vi "niRFUtil WFM Detect Multiple Bursts (real wfm).vi"(0 "Waveform In (Ohm Voltage)":T2 {"y" min=0 max=127 format="%.2f"; "dx" format="%^.2e"; "x0" format="%^.2e"}, 5 "Burst Detection Settings":T1={"Mode"=enum."Sliding Window", "Sliding Window Settings"={"Chunks"=500, "Threshold (dB)"=12.0}, "Threshold Settings"={"Threshold Level (dB)"=-50.0, "Minimum Quiet Time (s)"=0.0001, "Threshold Type"=enum."Absolute"}} {"Threshold Settings"."Minimum Quiet Time (s)" format="%.3p"; "Threshold Settings"."Threshold Level (dB)" format="%.3g"; "Sliding Window Settings"."Threshold (dB)" format="%.3g"}) -> (4 "Number of Bursts Detected":i32, 6 "Burst Positions":cluster{"Start (s)":dbl, "Duration (s)":dbl}[](array[cluster]) {"Start (s)" format="%^.3e"; "Duration (s)" format="%^.3e"})   [LabVIEW 2015, in "niRFUtil.lvlib"]
uses:
  niRFUtil.lvlib
  Includes/niRFUtil INC Real Waveform.ctl
  Includes/niRFUtil INC Real Array.ctl
  Includes/niRFUtil INC Edge Detection Settings.ctl
  Includes/niRFUtil INC Edge Type.ctl
  niRFUtil WFM Detect Edge (complex wfm).vi
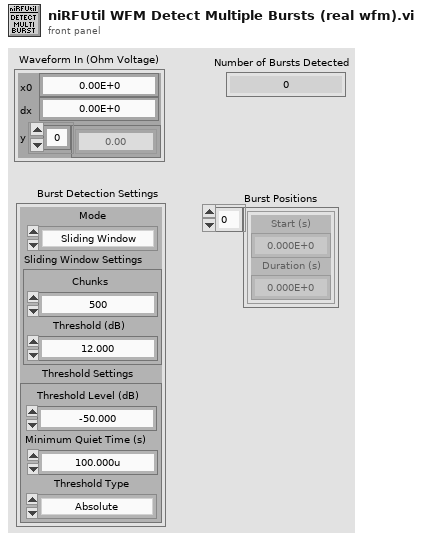
[diagram p1: front panel]
types:
  T1 = typedef "niRFUtil.lvlib/niRFUtil INC Edge Detection Settings.ctl" = cluster{"Mode":enum16{"Sliding Window", "Threshold"}, "Sliding Window Settings":cluster{"Chunks":i32, "Threshold (dB)":dbl}, "Threshold Settings":cluster{"Threshold Level (dB)":dbl, "Minimum Quiet Time (s)":dbl, "Threshold Type":enum16{"Relative", "Absolute"}}}
  T2 = typedef "niRFUtil.lvlib/niRFUtil INC Real Waveform.ctl" = cluster{"x0":dbl, "dx":dbl, "y":T3}
  T3 = typedef "niRFUtil.lvlib/niRFUtil INC Real Array.ctl" = sgl[]
  T4 = typedef "niRFUtil.lvlib/niRFUtil INC Edge Type.ctl" = enum16{"Rising", "Falling"}
  T5 = typedef "niRFUtil.lvlib/niRFUtil INC Complex Waveform.ctl" = cluster{"x0":dbl, "dx":dbl, "y":T6}
  T6 = typedef "niRFUtil.lvlib/niRFUtil INC Complex Array.ctl" = csg[]
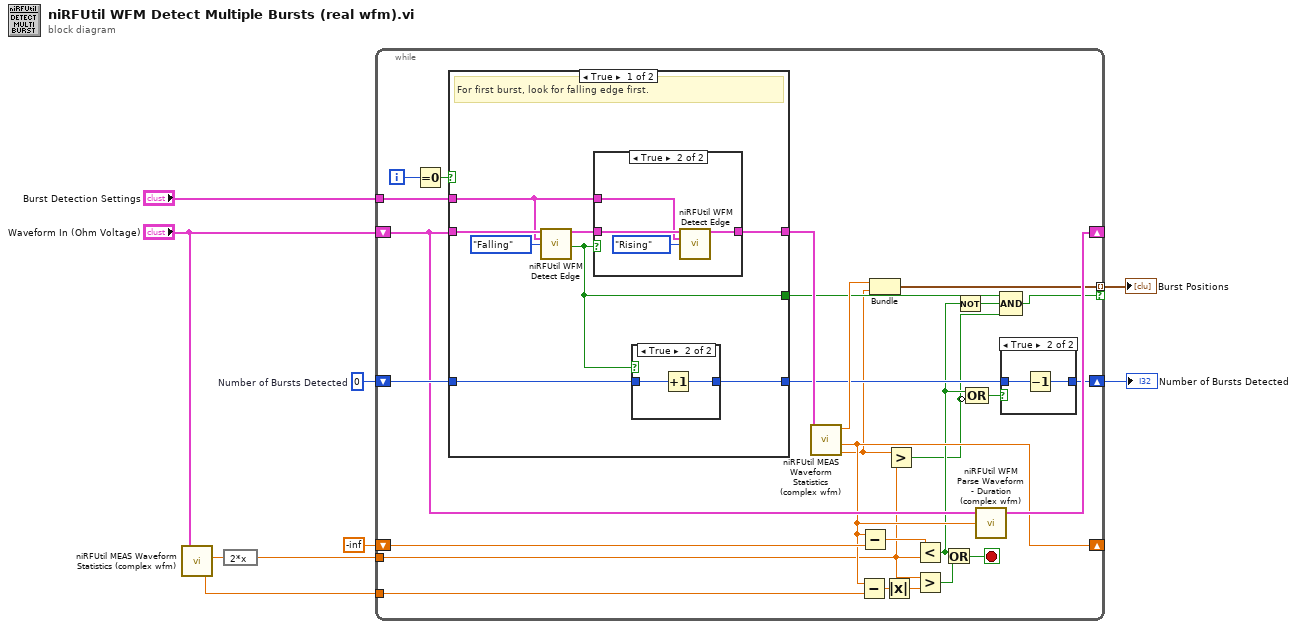
[diagram p0: block diagram]
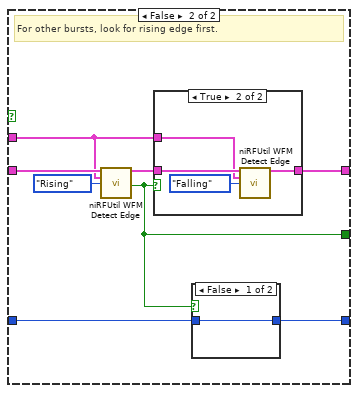
[diagram p5: hidden frame]
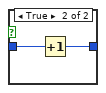
[diagram p6: hidden frame]
diagram:
  w9 = 0  # Number of Bursts Detected
  n1 = call "niRFUtil MEAS Waveform Statistics (complex wfm).vi"("Waveform In"="Waveform In (Ohm Voltage)") -> ("Interval"=w7:dbl, "End + Interval"=w5:dbl)  [unwired: 4 in, 2 out]
  n2 = expression code="2*x"(w7) -> (w6:dbl)
  n3 = while {
    shift-right: [w31] -> _
    shift-left: "Waveform In (Ohm Voltage)" -> [w33]
    shift-right: [w19] -> w4
    shift-left: w9 -> [w34]
    shift-right: [w22] -> _
    shift-left: -inf ("End") -> [w30]
    tunnel: w6 -> [w14]
    tunnel: w5 -> [w28]
    tunnel: [w21] -> w3 mode=indexing if=w16
    tunnel: "Burst Detection Settings" -> [w15]
    i -> [w36]
    stop <- w24 stop-if-true
    n4 = Equal To 0?(x=w36) -> (x = 0?=w35:bool)
    n5 = case shown="True" w35 {
      tunnel: w33 -> [w47 w63]
      tunnel: [w44 w60] -> w32
      tunnel: w34 -> [w43 w59]
      tunnel: [w42 w58] -> w20
      tunnel: [w41 w57] -> w17
      tunnel: w15 -> [w40 w56]
      frame True {
        # "For first burst, look for falling edge first."
        n6 = call-poly "niRFUtil WFM Detect Edge.vi"("Input Waveform"=w47, "Edge Detection Settings"=w40, "Edge Type"=niRFUtil_INC_Edge_Type."Falling") -> ("Output Waveform"=w45:T5, "Edge Detected?"=w41:bool)  [unwired: 9 in, 2 out]
        n7 = case shown="True" w41 {
          tunnel: w45 -> [w51 w55]
          tunnel: [w51 w53] -> w44
          tunnel: w40 -> [_ w52]
          frame False {
          }
          frame True {
            n8 = call-poly "niRFUtil WFM Detect Edge.vi"("Input Waveform"=w55, "Edge Detection Settings"=w52, "Edge Type"=niRFUtil_INC_Edge_Type."Rising") -> ("Output Waveform"=w53:T5)  [unwired: 9 in, 3 out]
          }
        }
        n9 = case shown="True" w41 {
          tunnel: w43 -> [w48 w50]
          tunnel: [w48 w49] -> w42
          frame False {
          }
          frame True {
            n10 = Increment(x=w50) -> (x+1=w49:i32)
          }
        }
      }
      frame False {
        # "For other bursts, look for rising edge first."
        n11 = call-poly "niRFUtil WFM Detect Edge.vi"("Input Waveform"=w63, "Edge Detection Settings"=w56, "Edge Type"=niRFUtil_INC_Edge_Type."Rising") -> ("Output Waveform"=w61:T5, "Edge Detected?"=w57:bool)  [unwired: 9 in, 2 out]
        n12 = case shown="True" w57 {
          tunnel: w61 -> [w67 w71]
          tunnel: [w67 w69] -> w60
          tunnel: w56 -> [_ w68]
          frame False {
          }
          frame True {
            n13 = call-poly "niRFUtil WFM Detect Edge.vi"("Input Waveform"=w71, "Edge Detection Settings"=w68, "Edge Type"=niRFUtil_INC_Edge_Type."Falling") -> ("Output Waveform"=w69:T5)  [unwired: 9 in, 3 out]
          }
        }
        n14 = case shown="False" w57 {
          tunnel: w59 -> [w64 w66]
          tunnel: [w64 w65] -> w58
          frame False {
          }
          frame True {
            n15 = Increment(x=w66) -> (x+1=w65:i32)
          }
        }
      }
    }
    n16 = call "niRFUtil MEAS Waveform Statistics (complex wfm).vi"("Waveform In"=w32) -> ("Start"=w23:dbl, "End + Interval"=w22:dbl, "Duration"=w10:dbl)  [unwired: 4 in, 1 out]
    n17 = Subtract(x=w22, y=w28) -> (x-y=w27:dbl)
    n18 = Subtract(x=w22, y=w30) -> (x-y=w29:dbl)
    n19 = Bundle("Start"=w23, "Duration"=w10) -> (w21:cluster{"Start":dbl, "Duration":dbl})  [unwired: 1 in]
    n20 = Absolute Value(x=w27) -> (abs(x)=w26:dbl)
    n21 = Greater?(x=w10, y=w14) -> (0:w11:bool)
    n22 = Less?(x=w29, y=w14) -> (x < y?=w13:bool)
    n23 = Greater?(x=w14, y=w26) -> (0:w25:bool)
    n24 = Or(x=w13, y=w25) -> (x .or. y?=w24:bool)
    n25 = Not(x=w13) -> (.not. x?=w18:bool)
    n26 = Compound Arithmetic op=OR(w13, invert w11) -> (w12:bool)
    n27 = call "niRFUtil WFM Parse Waveform - Duration (complex wfm).vi"("Start (-Inf)"=w22, "Waveform In"=w33) -> ("Waveform Out"=w31:T5)  [unwired: 3 in]
    n28 = Compound Arithmetic op=AND(w17, w18, w11) -> (w16:bool)
    n29 = case shown="True" w12 {
      tunnel: w20 -> [w37 w39]
      tunnel: [w37 w38] -> w19
      frame False {
      }
      frame True {
        n30 = Decrement(x=w39) -> (x-1=w38:i32)
      }
    }
  }
  "Number of Bursts Detected" <- w4
  "Burst Positions" <- w3
